vi "SetNofFFTLines.vi"(8 "error in (no error)":errorcluster, 9 "NofLines":i32, 10 "Analyzer (0: A0)":i32(ring) items=["A0", "A1"], 11 "VISA resource name":refnum<visa-resource-name>) -> (0 "error out":errorcluster, 3 "VISA resource name out":refnum<visa-resource-name>)   [LabVIEW 2014, in "Stanford Research SR1.lvlib"]
doc: "Sets the actual NofLines."
uses:
  Stanford Research SR1.lvlib
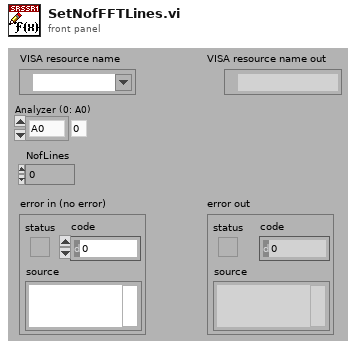
[diagram p1: front panel]
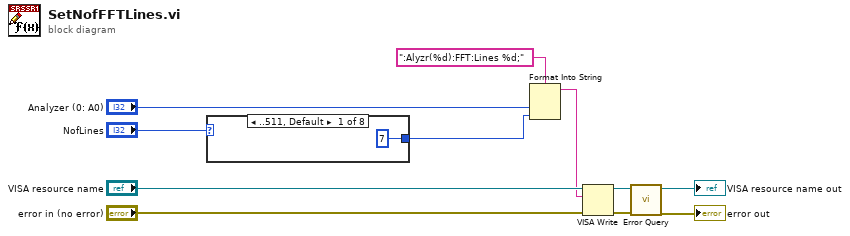
[diagram p0: block diagram]
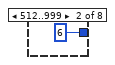
[diagram p2: hidden frame]
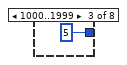
[diagram p3: hidden frame]
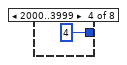
[diagram p4: hidden frame]
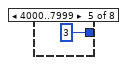
[diagram p5: hidden frame]
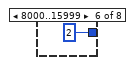
[diagram p6: hidden frame]
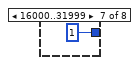
[diagram p7: hidden frame]
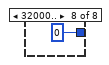
[diagram p8: hidden frame]
diagram:
  n1 = case shown="..511, Default" "NofLines" {
    tunnel: [7 6 5 4 3 2 1 0] -> w1
    frame ..511, Default {
    }
    frame 512..999 {
    }
    frame 1000..1999 {
    }
    frame 2000..3999 {
    }
    frame 4000..7999 {
    }
    frame 8000..15999 {
    }
    frame 16000..31999 {
    }
    frame 32000.. {
    }
  }
  n2 = Format Into String(format string=":Alyzr(%d):FFT:Lines %d;", "Analyzer (0: A0)", w1) -> (resulting string=w6:string)  [unwired: 2 in, 1 out]
  n3 = VISA Write(VISA resource name="VISA resource name", write buffer=w6, error in (no error)="error in (no error)") -> (VISA resource name out=w4:refnum<visa-resource-name>, error out=w3:errorcluster)  [unwired: 1 out]
  n4 = call "Error Query.vi"("error in (no error)"=w3, "VISA resource name"=w4) -> ("error out"=→"error out":errorcluster, "VISA resource name out"=→"VISA resource name out":refnum<visa-resource-name>)  [unwired: 6 in, 2 out]
